vi "GlueCustomLinePattern.vi"(10 "Stereo Angle [mrad]":dbl=-26.0 format="%#_13g", 11 "Calibration Directory":path) -> ()   [LabVIEW 2016]
uses:
  <vilib>/LabVIEW Interface for Arduino/Type Defs/Arduino Resource.ctl
  <vilib>/LabVIEW Interface for Arduino/Type Defs/Board Type.ctl
  <vilib>/LabVIEW Interface for Arduino/Type Defs/Pin Mode.ctl
  <vilib>/Utility/file.llb/Read Delimited Spreadsheet (DBL).vi
  <vilib>/LabVIEW Interface for Arduino/LabVIEW Interface for Arduino.lvlib
panel:
  in  "Lines Control":enum32{"Repeated Lines", "Custom Lines"}(tab)
  in  "Relative Line Separations [mm]":dbl[][](array[numeric])=[[10.0, 0.0], [7.5, 5.0], [5.0, 5.0], [5.0, 5.0], [5.0, 5.0], [5.0, 12.5], [5.0, 5.0], [5.0, 5.0], [5.0, 5.0], [5.0, 5.0], [5.0, 5.0], [5.0, 5.0], [5.0, 5.0], [5.0, 5.0], [5.0, 5.0], [5.0, 5.0], [15.0, 5.0]] format="%#_13g"
  in  "Line Widths [mm]":dbl[](array[numeric])=[60.0, 75.0, 75.0, 75.0, 75.0, 75.0, 75.0, 75.0, 75.0, 75.0, 75.0, 75.0, 75.0, 75.0, 75.0, 75.0, 37.5] format="%#_13g"
  in  "Line Speeds [mm/s]":dbl[][](array[numeric])=[[12.5, 12.5, 75.0, 75.0, 75.0, 75.0], [25.0, 25.0, 0.0, 0.0, 0.0, 0.0], [25.0, 25.0, 0.0, 0.0, 0.0, 0.0], [25.0, 25.0, 0.0, 0.0, 0.0, 0.0], [25.0, 25.0, 0.0, 0.0, 0.0, 0.0], [25.0, 25.0, 0.0, 0.0, 0.0, 0.0], [25.0, 25.0, 0.0, 0.0, 0.0, 0.0], [25.0, 25.0, 0.0, 0.0, 0.0, 0.0], [25.0, 25.0, 0.0, 0.0, 0.0, 0.0], [25.0, 25.0, 0.0, 0.0, 0.0, 0.0], [25.0, 25.0, 0.0, 0.0, 0.0, 0.0], [25.0, 25.0, 0.0, 0.0, 0.0, 0.0], [25.0, 25.0, 0.0, 0.0, 0.0, 0.0], [25.0, 25.0, 0.0, 0.0, 0.0, 0.0], [25.0, 25.0, 0.0, 0.0, 0.0, 0.0], [25.0, 25.0, 0.0, 0.0, 0.0, 0.0], [25.0, 25.0, 0.0, 0.0, 0.0, 0.0]] format="%#_13g"
  in  "AL - Left Start Relative to Corner [mm]":dbl[][](array[numeric])=[[62.5, 122.5], [-5.0, 35.0], [40.0, 35.0]]
  in  "AL - Line Widths [mm]":dbl[](array[numeric])=[10.0, 35.0, 35.0]
  in  "AL - Line Speeds [mm/s]":dbl[][](array[numeric])=[[5.0, 5.0, 0.0], [12.5, 12.5, 0.0], [12.5, 12.5, 0.0]]
  in  "Outputs Tab":T1(tab)
  out "Running Positions (Repeated) [mm]":dbl[][](array[numeric])
  out "Running Positions (Custom) [mm]":dbl[][](array[numeric])
  out "All Positions [mm]":dbl[][](array[numeric])
  in  "Inputs Tab":T2(tab)
  out "Virtual Stave Map":path
  out "Stave Angle [rad]":dbl format="%#_13g"
  out "Total Angle [rad]":dbl
  in  "Module Number":i32=7
  in  "Glue Additional Lines":bool
  out "Arduino Resource":T3={"VISA resource"="GlueCTRL", "Board Type"=enum."Uno", "Connection Type"=enum."USB / Serial", "Bytes Per Packet (15)"=15}
  in  "Digital I/O Pin":u8=7
  in  "Default Axis Speeds":T5={"X [mm/s]"=25.0, "Y [mm/s]"=25.0, "Z [mm/s]"=25.0}
  in  "Pause After Gluing [ms]":dbl=250.0 format="%#_13g"
  out "N Lines (Repeated)":i32
  out "N Lines (Custom)":i32
  in  "Fine Axis Speeds":T5={"X [mm/s]"=25.0, "Y [mm/s]"=25.0, "Z [mm/s]"=25.0}
  in  "Positions [mm]":dbl[][](array[numeric])
  in  "OK Button":bool
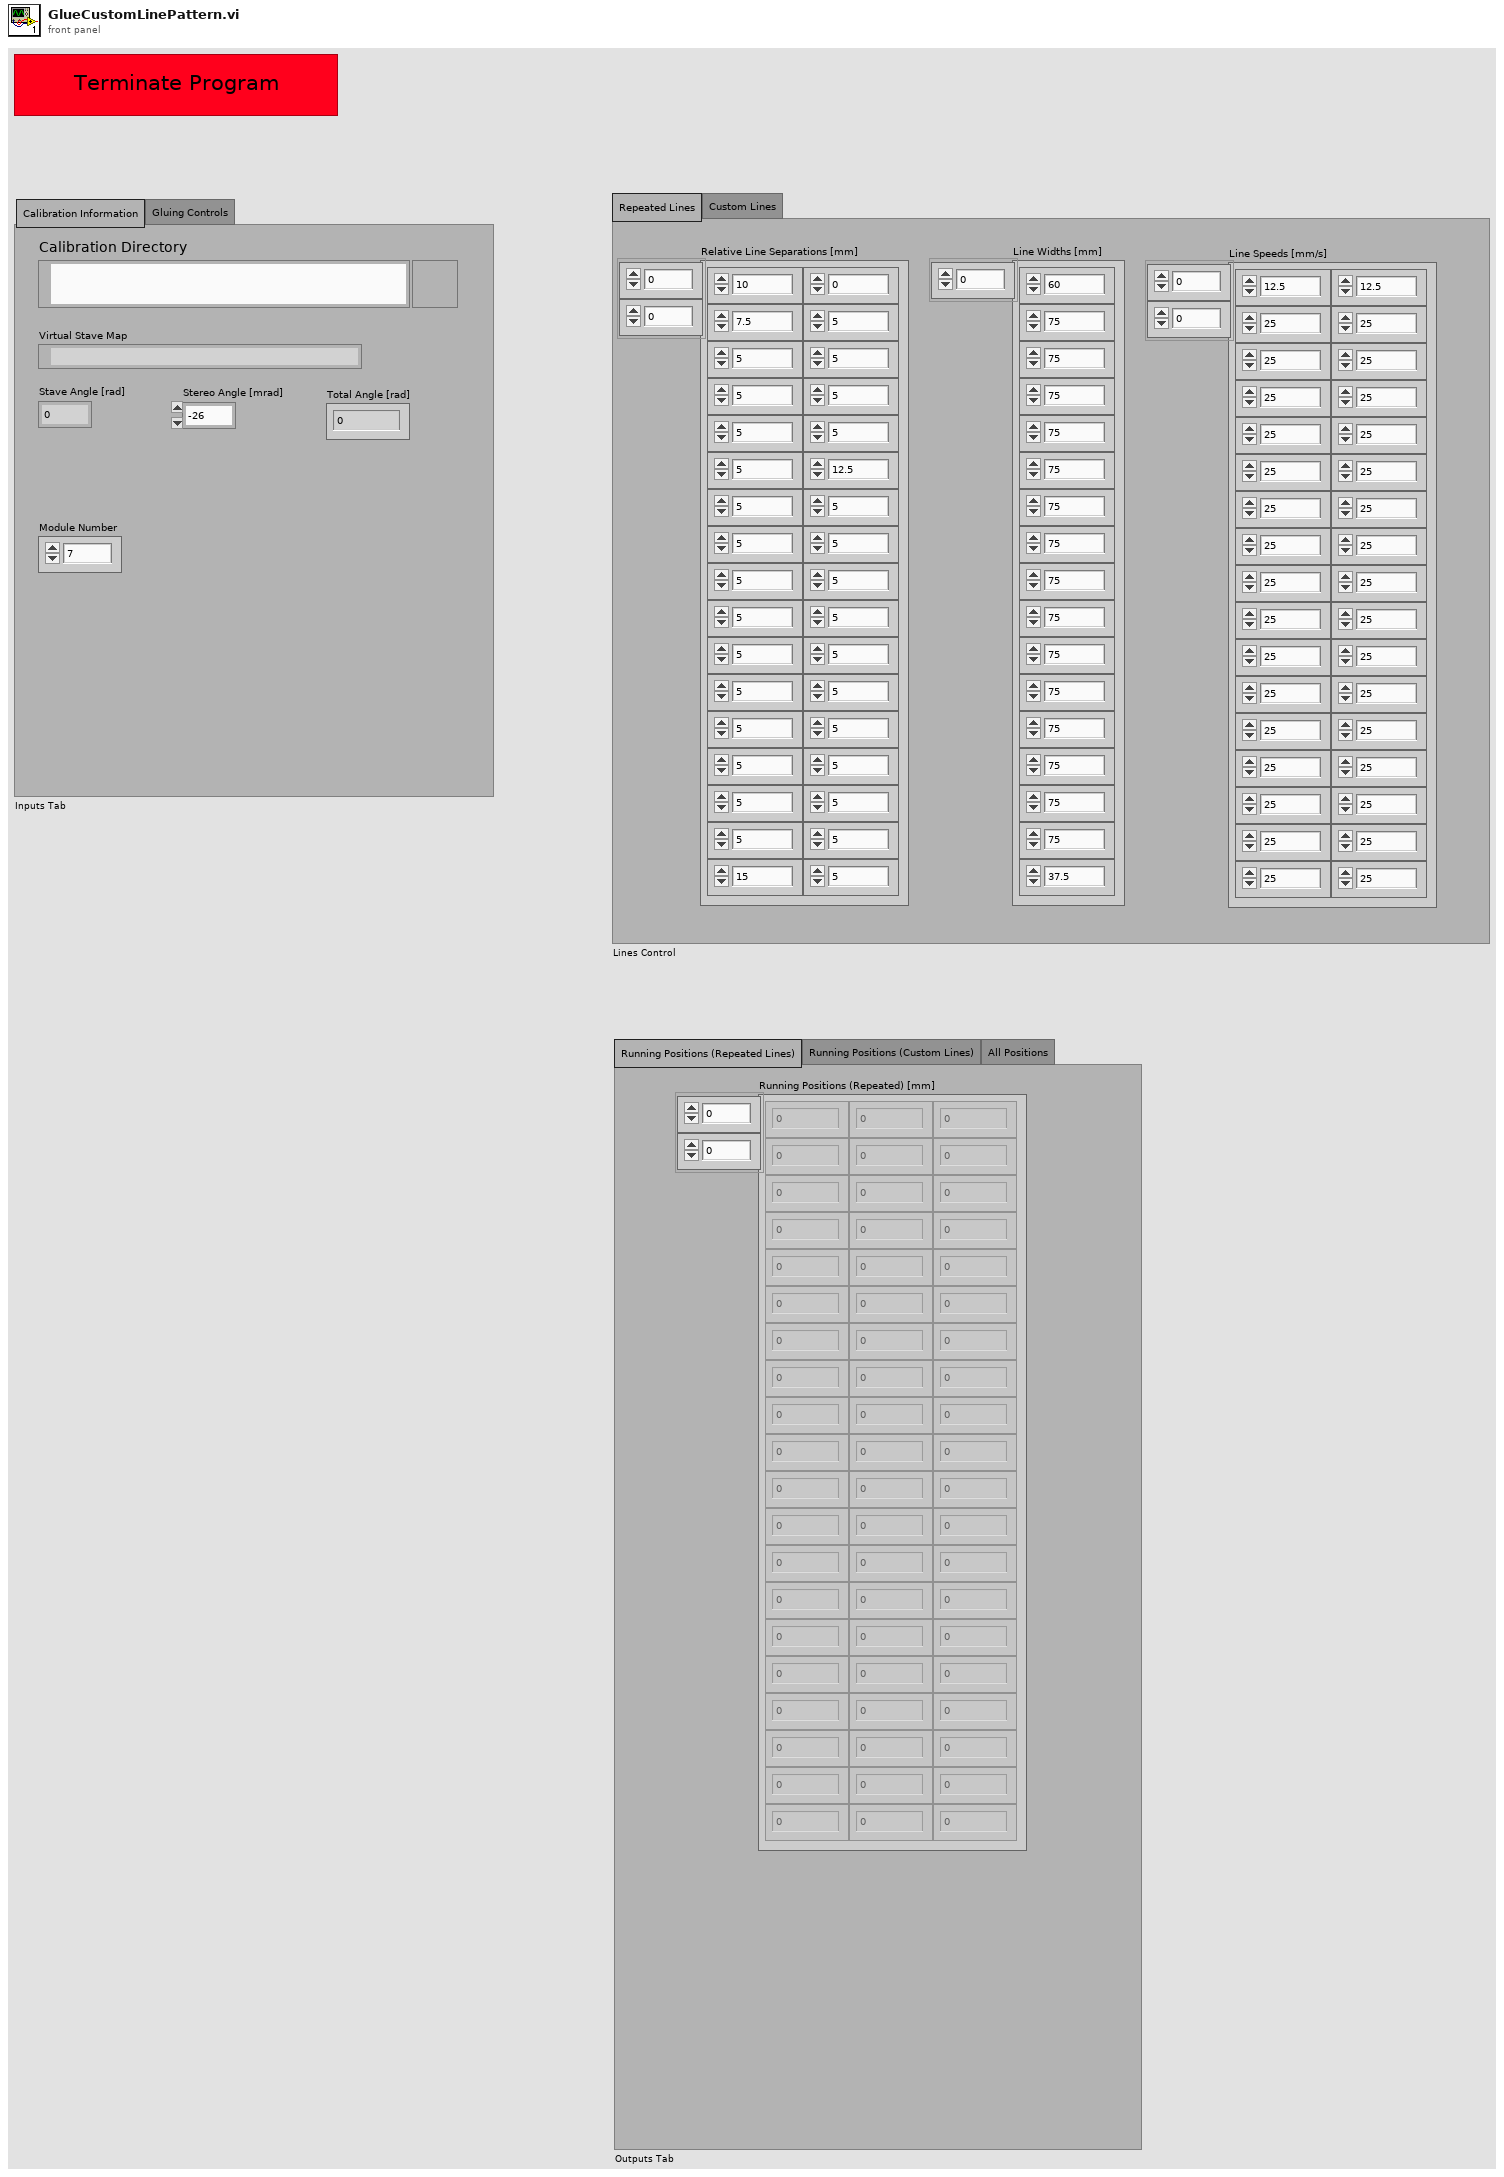
[diagram p1: front panel]
types:
  T1 = enum32{"Running Positions (Repeated Lines)", "Running Positions (Custom Lines)", "All Positions"}
  T2 = enum32{"Calibration Information", "Gluing Controls"}
  T3 = typedef "LabVIEW Interface for Arduino.lvlib/Arduino Resource.ctl" = cluster{"VISA resource":refnum<visa-resource-name>, "Board Type":T4, "Connection Type":enum8{"USB / Serial"}, "Bytes Per Packet (15)":u8}
  T4 = typedef "LabVIEW Interface for Arduino.lvlib/Board Type.ctl" = enum16{"Uno", "Dimuelanove w/Atmega 328", "Mega 2560"}
  T5 = cluster{"X [mm/s]":dbl, "Y [mm/s]":dbl, "Z [mm/s]":dbl}
  T6 = typedef "LabVIEW Interface for Arduino.lvlib/Pin Mode.ctl" = enum8{"Input", "Output"}
  T7 = cluster{"Final X":dbl, "Final Y":dbl, "Final Z":dbl}
  T8 = cluster{"Line Separation [mm]":dbl, "Line Separation [mm]":dbl, "Z [mm/s]":dbl}
  T9 = cluster{"Numeric Control":dbl, "Numeric Control":dbl, "Z [mm/s]":dbl}
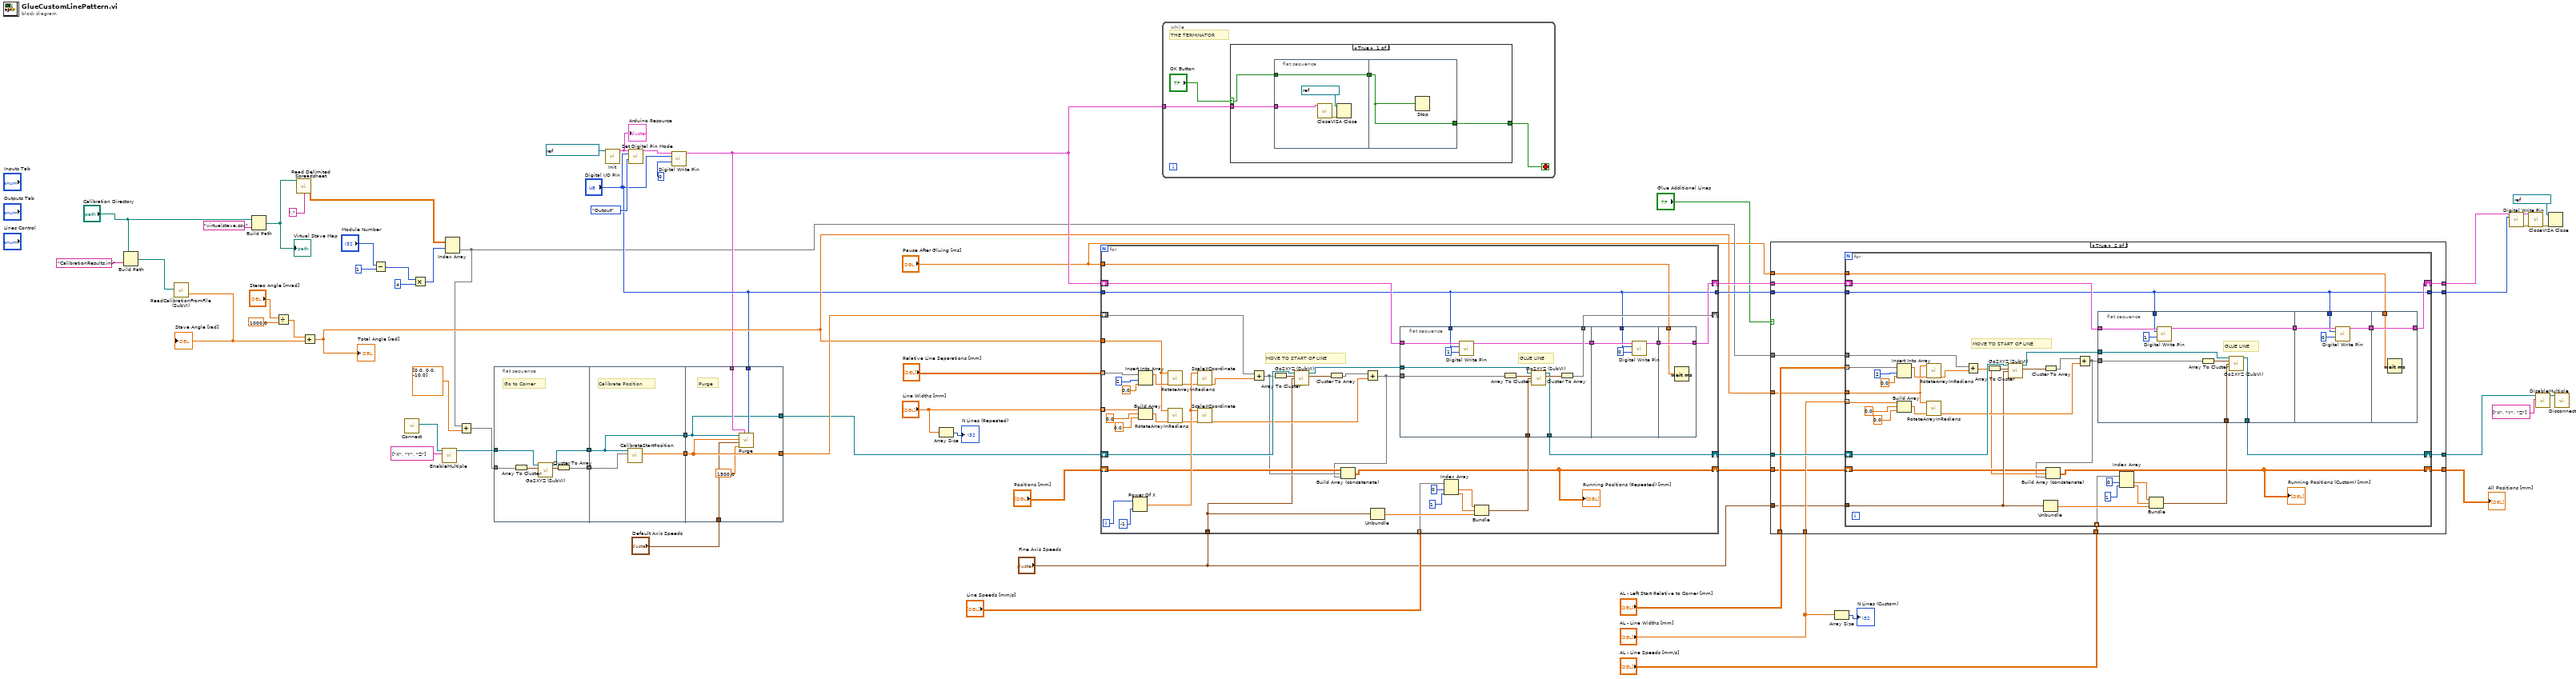
[diagram p0: block diagram]
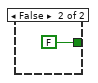
[diagram p3: hidden frame]
diagram:
  n1 = Build Path(base path="Calibration Directory", name or relative path="CalibrationResults.ini") -> (appended path=w57:path)
  n2 = call "ReadCalibrationFromFile (SubVI).vi"("Calibration file path"=w57) -> ("Angle"=w54:dbl)  [unwired: 12 in, 6 out]
  "Stave Angle [rad]" <- w54
  n3 = Build Path(base path="Calibration Directory", name or relative path="virtualstave.csv") -> (appended path=w62:path)
  "Virtual Stave Map" <- w62
  n4 = Divide(x="Stereo Angle [mrad]", y=1000.0) -> (x/y=w53:dbl)
  n5 = call-poly <vilib>:"Read Delimited Spreadsheet.vi"("file path (dialog if empty)"=w62, "delimiter (\\t)"="," ("delimiter (\\t)")) -> ("all rows"=w58:dbl[][])  [unwired: 8 in, 5 out]
  n6 = Add(x=w53, y=w54) -> (x+y=w17:dbl)
  "Total Angle [rad]" <- w17
  n7 = Subtract(x="Module Number", y=1) -> (x-y=w59:i32)
  n8 = call "Connect.vi"() -> ("controller"=w49:refnum<k24>)  [unwired: 10 in, 1 out]
  n9 = Multiply(x=w59, y=4) -> (x*y=w60:i32)
  n10 = call "EnableMultiple.vi"("axis names"=string[] ["X", "Y", "Z"] ("Axes Names"), "controller in"=w49) -> ("controller out"=w16:refnum<k24>)  [unwired: 8 in, 1 out]
  n11 = Index Array(array=w58, index (row)=w60) -> (element=w6:dbl[])  [unwired: 1 in]
  n12 = Add(x=w6, y=dbl[] [0.0, 0.0, -10.0]) -> (x+y=w4:dbl[])
  n13 = flat-sequence {
    tunnel: w16 -> [w67]
    tunnel: [w66] -> w15
    tunnel: w4 -> [w65]
    tunnel: [w64] -> w14
    tunnel: w15 -> [w71]
    tunnel: w14 -> [w72]
    tunnel: [w71] -> w13
    tunnel: [w70] -> w12
    tunnel: w13 -> [w74]
    tunnel: w12 -> [w78]
    tunnel: [w78] -> w11
    tunnel: "Default Axis Speeds" -> [w77]
    tunnel: "Digital I/O Pin" -> [w76]
    tunnel: w8 -> [w75]
    tunnel: [w74] -> w7
    frame #0 {
      # "Go to Corner"
      n14 = Array To Cluster(array=w65) -> (cluster=w69:cluster{"[0]":dbl, "[1]":dbl, "[2]":dbl})
      n15 = call "Go2XYZ (SubVI).vi"(".NET Refnum in"=w67, "Go to Coordinates"=w69) -> (".NET Refnum out"=w66:refnum<k24>, "Final Position"=w68:T7)  [unwired: 9 in, 3 out]
      n16 = Cluster To Array(cluster=w68) -> (array=w64:dbl[])
    }
    frame #1 {
      # "Calibrate Position"
      n17 = call "CalibrateStartPosition.vi"("Start Position [mm]"=w72, ".NET Refnum In"=w71) -> ("Final Position [mm]"=w70:dbl[])  [unwired: 9 in]
    }
    frame #2 {
      # "Purge"
      n18 = call "Purge.vi"("Digital I/O Pin"=w76, "Arduino Resource"=w75, "Purge Time [ms]"=1500.0, "Axis Speeds"=w77, "Start Position [mm]"=w78, ".NET Refnum In"=w74) -> ()  [unwired: 6 in]
    }
  }
  n19 = call <vilib>:"Init.vi"("VISA resource"=refnum<visa-resource-name> "GlueCTRL") -> ("Arduino Resource"=w43:T3)  [unwired: 17 in, 1 out]
  "Arduino Resource" <- w43
  n20 = call <vilib>:"Set Digital Pin Mode.vi"("Arduino Resource"=w43, "Digital I/O Pin"="Digital I/O Pin", "Pin Mode (Input)"=Pin_Mode."Output") -> ("Arduino Resource"=w46:T3)  [unwired: 11 in, 1 out]
  n21 = call <vilib>:"Digital Write Pin.vi"("Arduino Resource"=w46, "Digital I/O Pin (0)"="Digital I/O Pin", "Value (0)"=u8 0) -> ("Arduino Resource"=w8:T3)  [unwired: 11 in, 1 out]
  n22 = Array Size(array="Line Widths [mm]") -> (size(s)=→"N Lines (Repeated)":i32)
  n23 = for {
    tunnel: "Relative Line Separations [mm]" -> [w116] mode=indexing
    tunnel: "Line Widths [mm]" -> [w117] mode=indexing
    tunnel: w17 -> [w111]
    shift-right: [w102] -> _
    shift-left: w11 -> [w106]
    tunnel: "Line Speeds [mm/s]" -> [w99] mode=indexing
    shift-right: [w94] -> w28
    shift-left: w7 -> [w93]
    shift-right: [w89] -> w26
    shift-left: w8 -> [w91]
    shift-right: [w82] -> w21
    shift-left: "Positions [mm]" -> [w86]
    tunnel: "Digital I/O Pin" -> [w88]
    tunnel: [w88] -> w24
    tunnel: "Pause After Gluing [ms]" -> [w80]
    tunnel: "Fine Axis Speeds" -> [w79]
    i -> [w85]
    # "MOVE TO START OF LINE"
    n24 = Power Of X(1:-1 ("x"), 2:w85) -> (0:w109:dbl)
    n25 = Insert Into Array(array=w116, index=2, new element=0.0 ("new element/subarray")) -> (w113:dbl[])
    n26 = Build Array(w117, 0.0 ("element"), 0.0 ("element")) -> (w112:dbl[])
    n27 = call "RotateArrayInRadians.vi"("X,Y,Z Input"=w113, "Angle"=w111) -> ("X,Y,Z Output"=w107:dbl[])  [unwired: 9 in]
    n28 = call "RotateArrayInRadians.vi"("X,Y,Z Input"=w112, "Angle"=w111) -> ("X,Y,Z Output"=w108:dbl[])  [unwired: 9 in]
    n29 = call "ScaleXCoordinate.vi"("X, Y, Z Input"=w107, "Scale"=w109) -> ("-X, Y, Z Output"=w104:dbl[])  [unwired: 9 in]
    n30 = call "ScaleXCoordinate.vi"("X, Y, Z Input"=w108, "Scale"=w109) -> ("-X, Y, Z Output"=w87:dbl[])  [unwired: 9 in]
    n31 = Add(x=w106, y=w104) -> (x+y=w84:dbl[])
    n32 = Array To Cluster(array=w84) -> (cluster=w105:cluster{"[0]":dbl, "[1]":dbl, "[2]":dbl})
    n33 = call "Go2XYZ (SubVI).vi"(".NET Refnum in"=w93, "Go to Coordinates"=w105, "Axis Speeds"=w79) -> (".NET Refnum out"=w103:refnum<k24>, "Final Position"=w110:T7)  [unwired: 8 in, 3 out]
    n34 = Cluster To Array(cluster=w110) -> (array=w92:dbl[])
    n35 = Add(x=w92, y=w87) -> (x+y=w83:dbl[])
    n36 = Build Array (concatenate)(w86, w84, w83) -> (w82:dbl[][])
    "Running Positions (Repeated) [mm]" <- w82
    n37 = Unbundle(w79) -> ("Z [mm/s]"=w101:dbl)  [unwired: 2 out]
    n38 = flat-sequence {
      tunnel: [w127] -> w102
      tunnel: w100 -> [w126]
      tunnel: [w125] -> w94
      tunnel: [w124] -> w90
      tunnel: w88 -> [w122]
      tunnel: w91 -> [w123]
      tunnel: w103 -> [w128]
      tunnel: w83 -> [w130]
      tunnel: w90 -> [w135]
      tunnel: w88 -> [w133]
      tunnel: [w134] -> w81
      tunnel: [w137] -> w89
      tunnel: w81 -> [w137]
      tunnel: w80 -> [w136]
      frame #0 {
        # "GLUE LINE"
        n39 = call <vilib>:"Digital Write Pin.vi"("Arduino Resource"=w123, "Digital I/O Pin (0)"=w122, "Value (0)"=u8 1) -> ("Arduino Resource"=w124:T3)  [unwired: 11 in, 1 out]
        n40 = Array To Cluster(array=w130) -> (cluster=w129:cluster{"[0]":dbl, "[1]":dbl, "[2]":dbl})
        n41 = call "Go2XYZ (SubVI).vi"(".NET Refnum in"=w128, "Go to Coordinates"=w129, "Axis Speeds"=w126) -> (".NET Refnum out"=w125:refnum<k24>, "Final Position"=w131:T7)  [unwired: 8 in, 3 out]
        n42 = Cluster To Array(cluster=w131) -> (array=w127:dbl[])
      }
      frame #1 {
        n43 = call <vilib>:"Digital Write Pin.vi"("Arduino Resource"=w135, "Digital I/O Pin (0)"=w133, "Value (0)"=u8 0) -> ("Arduino Resource"=w134:T3)  [unwired: 11 in, 1 out]
      }
      frame #2 {
        n44 = Wait (ms)(milliseconds to wait=w136) -> ()  [unwired: 1 out]
      }
    }
    n45 = Index Array(array=w99, index #1=0 ("index"), index #2=1 ("index")) -> (element #1=w95:dbl, element #2=w96:dbl)
    n46 = Bundle("Line Separation [mm]"=w95, "Line Separation [mm]"=w96, "Z [mm/s]"=w101) -> (w100:T8)  [unwired: 1 in]
  }
  n47 = while {
    tunnel: w8 -> [w139]
    stop <- w138 stop-if-true
    # "THE TERMINATOR"
    n48 = case shown="True" "OK Button" {
      selector: "OK Button" -> [w144 _]
      tunnel: w139 -> [w142 _]
      tunnel: [w141 FALSE] -> w138
      frame True {
        n49 = flat-sequence {
          tunnel: w144 -> [w146]
          tunnel: [w146] -> w143
          tunnel: w142 -> [w145]
          tunnel: w143 -> [w149]
          tunnel: [w149] -> w141
          frame #0 {
            n50 = call <vilib>:"Close.vi"("Arduino Resource"=w145) -> ("error out"=w147:errorcluster)  [unwired: 14 in]
            n51 = VISA Close(VISA resource name=refnum<visa-resource-name> "GlueCTRL", error in (no error)=w147) -> ()  [unwired: 1 out]
          }
          frame #1 {
            n52 = Stop(stop? (T)=w149) -> ()
          }
        }
      }
      frame False {
      }
    }
  }
  n53 = case shown="True" "Glue Additional Lines" {
    tunnel: "AL - Left Start Relative to Corner [mm]" -> [_ w164]
    tunnel: "AL - Line Widths [mm]" -> [_ w163]
    tunnel: "AL - Line Speeds [mm/s]" -> [_ w162]
    tunnel: w28 -> [w154 w169]
    tunnel: [w154 w168] -> w27
    tunnel: w26 -> [w153 w167]
    tunnel: [w153 w166] -> w25
    tunnel: w24 -> [w152 w165]
    tunnel: [w152 w161] -> w23
    tunnel: w17 -> [_ w160]
    tunnel: w6 -> [_ w158]
    tunnel: "Fine Axis Speeds" -> [_ w159]
    tunnel: w21 -> [w151 w157]
    tunnel: [w151 w156] -> w20
    tunnel: "Pause After Gluing [ms]" -> [_ w155]
    frame False {
    }
    frame True {
      n54 = for {
        shift-right: [w189] -> w168
        shift-left: w169 -> [w192]
        shift-right: [w187] -> w166
        shift-left: w167 -> [w188]
        tunnel: w164 -> [w199] mode=indexing
        tunnel: w163 -> [w198] mode=indexing
        tunnel: w162 -> [w178] mode=indexing
        tunnel: w160 -> [w197]
        tunnel: w159 -> [w179]
        tunnel: w158 -> [w176]
        shift-right: [w173] -> w156
        shift-left: w157 -> [w175]
        tunnel: w165 -> [w185]
        tunnel: [w185] -> w161
        tunnel: w155 -> [w170]
        # "MOVE TO START OF LINE"
        n55 = Insert Into Array(array=w199, index=2, new element=0.0 ("new element/subarray")) -> (w201:dbl[])
        n56 = Build Array(w198, 0.0 ("element"), 0.0 ("element")) -> (w200:dbl[])
        n57 = call "RotateArrayInRadians.vi"("X,Y,Z Input"=w201, "Angle"=w197) -> ("X,Y,Z Output"=w193:dbl[])  [unwired: 9 in]
        n58 = call "RotateArrayInRadians.vi"("X,Y,Z Input"=w200, "Angle"=w197) -> ("X,Y,Z Output"=w191:dbl[])  [unwired: 9 in]
        n59 = Add(x=w176, y=w193) -> (x+y=w174:dbl[])
        n60 = Array To Cluster(array=w174) -> (cluster=w195:cluster{"[0]":dbl, "[1]":dbl, "[2]":dbl})
        n61 = call "Go2XYZ (SubVI).vi"(".NET Refnum in"=w192, "Go to Coordinates"=w195, "Axis Speeds"=w179) -> (".NET Refnum out"=w186:refnum<k24>, "Final Position"=w196:T7)  [unwired: 8 in, 3 out]
        n62 = Unbundle(w179) -> ("Z [mm/s]"=w184:dbl)  [unwired: 2 out]
        n63 = Cluster To Array(cluster=w196) -> (array=w194:dbl[])
        n64 = Add(x=w194, y=w191) -> (x+y=w172:dbl[])
        n65 = Build Array (concatenate)(w175, w174, w172) -> (w173:dbl[][])
        "Running Positions (Custom) [mm]" <- w173
        n66 = flat-sequence {
          tunnel: [w214] -> w190
          tunnel: [w212] -> w189
          tunnel: w188 -> [w211]
          tunnel: w186 -> [w210]
          tunnel: w172 -> [w209]
          tunnel: w185 -> [w207]
          tunnel: w177 -> [w206]
          tunnel: w190 -> [w218]
          tunnel: w185 -> [w215]
          tunnel: [w217] -> w171
          tunnel: [w220] -> w187
          tunnel: w171 -> [w220]
          tunnel: w170 -> [w219]
          frame #0 {
            # "GLUE LINE"
            n67 = call <vilib>:"Digital Write Pin.vi"("Arduino Resource"=w211, "Digital I/O Pin (0)"=w207, "Value (0)"=u8 1) -> ("Arduino Resource"=w214:T3)  [unwired: 11 in, 1 out]
            n68 = Array To Cluster(array=w209) -> (cluster=w208:cluster{"[0]":dbl, "[1]":dbl, "[2]":dbl})
            n69 = call "Go2XYZ (SubVI).vi"(".NET Refnum in"=w210, "Go to Coordinates"=w208, "Axis Speeds"=w206) -> (".NET Refnum out"=w212:refnum<k24>)  [unwired: 8 in, 4 out]
          }
          frame #1 {
            n70 = call <vilib>:"Digital Write Pin.vi"("Arduino Resource"=w218, "Digital I/O Pin (0)"=w215, "Value (0)"=u8 0) -> ("Arduino Resource"=w217:T3)  [unwired: 11 in, 1 out]
          }
          frame #2 {
            n71 = Wait (ms)(milliseconds to wait=w219) -> ()  [unwired: 1 out]
          }
        }
        n72 = Index Array(array=w178, index #1=0 ("index"), index #2=1 ("index")) -> (element #1=w180:dbl, element #2=w181:dbl)
        n73 = Bundle("Numeric Control"=w180, "Numeric Control"=w181, "Z [mm/s]"=w184) -> (w177:T9)  [unwired: 1 in]
      }
    }
  }
  "All Positions [mm]" <- w20
  n74 = Array Size(array="AL - Line Widths [mm]") -> (size(s)=→"N Lines (Custom)":i32)
  n75 = call <vilib>:"Digital Write Pin.vi"("Arduino Resource"=w25, "Digital I/O Pin (0)"=w23) -> ("Arduino Resource"=w41:T3, "error out"=w40:errorcluster)  [unwired: 12 in]
  n76 = call <vilib>:"Close.vi"("Arduino Resource"=w41, "error in"=w40) -> ("error out"=w39:errorcluster)  [unwired: 13 in]
  n77 = call "DisableMultiple.vi"("axis names"=string[] ["X", "Y", "Z"], "controller in"=w27) -> ("controller out"=w38:refnum<k24>)  [unwired: 8 in, 1 out]
  n78 = VISA Close(VISA resource name=refnum<visa-resource-name> "GlueCTRL", error in (no error)=w39) -> ()  [unwired: 1 out]
  n79 = call "Disconnect.vi"("controller"=w38) -> ()  [unwired: 10 in, 1 out]
